vi "SolveMotor_Volts,Torque.vi"(8 "Reference Voltage (12)":dbl=12.0, 9 "Motor Characteristics":T2, 10 "Motor Torque":dbl, 11 "Motor Voltage":dbl) -> (3 "Motor Data":T1)   [LabVIEW 2014]
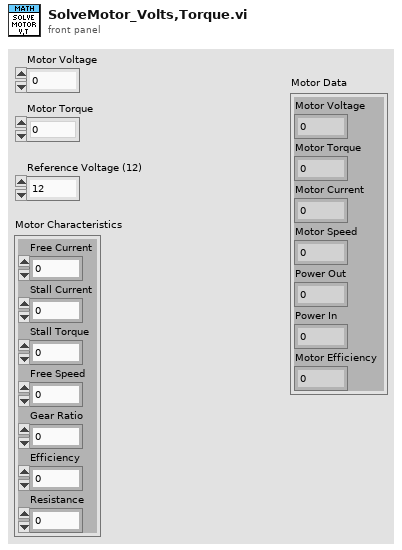
[diagram p1: front panel]
types:
  T1 = cluster{"Motor Voltage":dbl, "Motor Torque":dbl, "Motor Current":dbl, "Motor Speed":dbl, "Power Out":dbl, "Power In":dbl, "Motor Efficiency":dbl}
  T2 = cluster{"Free Current":dbl, "Stall Current":dbl, "Stall Torque":dbl, "Free Speed":dbl, "Gear Ratio":dbl, "Efficiency":dbl, "Resistance":dbl}
  T3 = cluster{"[0]":dbl, "[1]":dbl, "[2]":dbl, "[3]":dbl, "[4]":dbl, "[5]":dbl, "[6]":dbl}
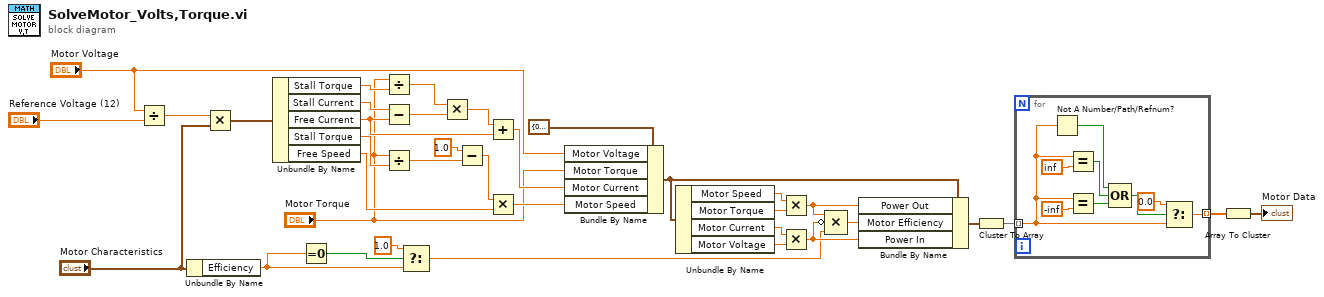
[diagram p0: block diagram]
diagram:
  n1 = Divide(x="Motor Voltage", y="Reference Voltage (12)") -> (x/y=w35:dbl)
  n2 = Unbundle By Name("Motor Characteristics") -> ("Efficiency"=w6:dbl)
  n3 = Multiply(x=w35, y="Motor Characteristics") -> (x*y=w34:T2)
  n4 = Unbundle By Name(w34) -> ("Stall Torque"=w33:dbl, "Stall Current"=w32:dbl, "Free Current"=w26:dbl, "Stall Torque"=w24:dbl, "Free Speed"=w22:dbl)
  n5 = Equal To 0?(x=w6) -> (x = 0?=w7:bool)
  n6 = Divide(x="Motor Torque", y=w33) -> (x/y=w30:dbl)
  n7 = Subtract(x=w32, y=w26) -> (x-y=w31:dbl)
  n8 = Divide(x="Motor Torque", y=w24) -> (x/y=w2:dbl)
  n9 = Select(t=1.0, s=w7, f=w6) -> (s? t:f=w4:dbl)
  n10 = Multiply(x=w30, y=w31) -> (x*y=w29:dbl)
  n11 = Subtract(x=1.0, y=w2) -> (x-y=w1:dbl)
  n12 = Add(x=w29, y=w26) -> (x+y=w27:dbl)
  n13 = Multiply(x=w1, y=w22) -> (x*y=w23:dbl)
  n14 = Bundle By Name(cluster=T1 {"Motor Voltage"=0.0, "Motor Torque"=0.0, "Motor Current"=0.0, "Motor Speed"=0.0, "Power Out"=0.0, "Power In"=0.0, "Motor Efficiency"=0.0} ("Motor Data"), "Motor Voltage"="Motor Voltage", "Motor Torque"="Motor Torque", "Motor Current"=w27, "Motor Speed"=w23) -> (w16:T1)
  n15 = Unbundle By Name(w16) -> ("Motor Speed"=w20:dbl, "Motor Torque"=w19:dbl, "Motor Current"=w17:dbl, "Motor Voltage"=w18:dbl)
  n16 = Multiply(x=w20, y=w19) -> (x*y=w14:dbl)
  n17 = Multiply(x=w17, y=w18) -> (x*y=w13:dbl)
  n18 = Compound Arithmetic op=MULTIPLY(w14, invert w13, w4) -> (w15:dbl)
  n19 = Bundle By Name(cluster=w16, "Power Out"=w14, "Motor Efficiency"=w15, "Power In"=w13) -> (w11:T1)
  n20 = Cluster To Array(cluster=w11) -> (array=w10:dbl[])
  n21 = for {
    tunnel: w10 -> [w42] mode=indexing
    tunnel: [w37] -> w9 mode=indexing
    n22 = Not A Number/Path/Refnum?(number/path/refnum=w42) -> (NaN/Path/Refnum?=w41:bool)
    n23 = Equal?(x=w42, y=inf) -> (x = y?=w39:bool)
    n24 = Equal?(x=w42, y=-inf) -> (x = y?=w40:bool)
    n25 = Compound Arithmetic op=OR(w41, w39, w40) -> (w38:bool)
    n26 = Select(t=0.0, s=w38, f=w42) -> (s? t:f=w37:dbl)
  }
  n27 = Array To Cluster(array=w9) -> (cluster=→"Motor Data":T3)
